vi "Get Morphology Structuring Element (Cross).vi"(7 "Anchor (Default: -1, -1 Use Centre)":T1={"x"=-1, "y"=-1}, 8 "error in (no error)":errorcluster, 11 "Size":T2) -> (0 "error out":errorcluster, 3 "Structuring Element":bool[][](array[boolean]))   [LabVIEW 2020, in "g_ar_toolkit.image.lvlib"]
uses:
  g_ar_toolkit.image.lvlib
  g_ar_toolkit.common/Image Size (Integer).ctl
  g_ar_toolkit.common/Image Point (Integer).ctl
  MorphologyStructuredElementShape.ctl
  g_ar_toolkit.common/Module Path.vi
  <vilib>/Utility/error.llb/Error Cluster From Error Code.vi
  g_ar_toolkit.common/g_ar_toolkit.common.lvlib
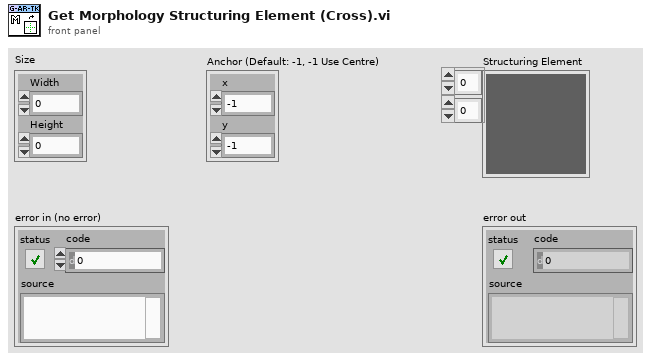
[diagram p1: front panel]
types:
  T1 = typedef "g_ar_toolkit.common.lvlib/Image Point (Integer).ctl" = cluster{"x":i32, "y":i32}
  T2 = typedef "g_ar_toolkit.common.lvlib/Image Size (Integer).ctl" = cluster{"Width":u16, "Height":u16}
  T3 = typedef "g_ar_toolkit.image.lvlib/MorphologyStructuredElementShape.ctl" = enum16{"Rect", "Cross", "Elipse"}
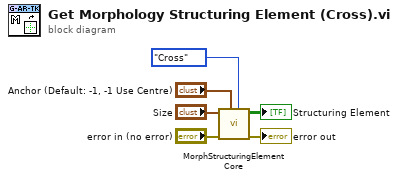
[diagram p0: block diagram]
diagram:
  n1 = call "MorphStructuringElementCore.vi"("Shape"=MorphologyStructuredElementShape."Cross", "Anchor (Default: -1, -1 Use Centre)"="Anchor (Default: -1, -1 Use Centre)", "error in (no error)"="error in (no error)", "Size"="Size") -> ("error out"=→"error out":errorcluster, "Structuring Element"=→"Structuring Element":bool[][])  [unwired: 6 in]
